vi "Delete Room.vi"(8 "error in (no error)":errorcluster, 10 "Room GUID":string, 11 "Room-API in":refnum<class "Room-API.lvclass">) -> (0 "error out":errorcluster, 2 "deleted?":bool, 3 "Room-API out":refnum<class "Room-API.lvclass">)   [LabVIEW 2020, in "Room-API.lvclass"]
uses:
  Room-API.lvclass
  Room-API.lvclass/Room-API.ctl
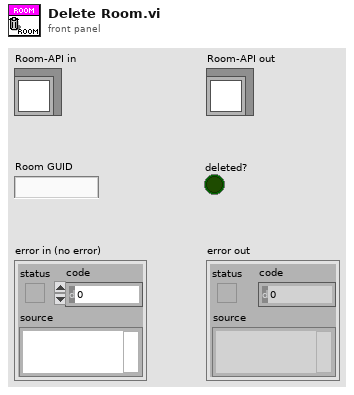
[diagram p1: front panel]
types:
  T1 = typedef "Room-API.lvclass/Single Room.ctl" = cluster{"name":string, "temperature_humidity":string[], "bond":string[], "hue":string[]}
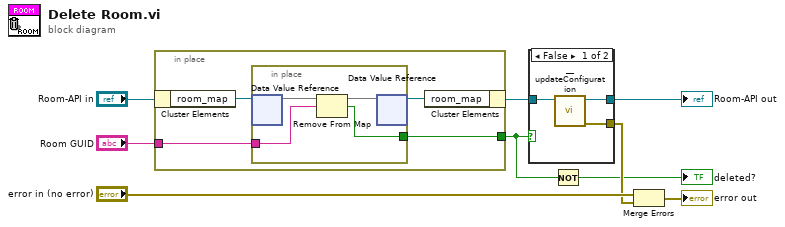
[diagram p0: block diagram]
diagram:
  n1 = in-place {
    in-place-border: "Room GUID" -> [w12]
    in-place-border: [w10] -> w2
    n2 = in-place-cluster #1("Room-API in") -> ("room_map"=w13:refnum<data-value>)
    n3 = in-place {
      in-place-border: w12 -> [w16]
      in-place-border: [w14] -> w10
      n4 = in-place-dvr #2(w13) -> (w17:map{string, T1})  [unwired: 1 out]
      n5 = Remove From Map(10:w16, 11:w17) -> (2:w14:bool, 3:w15:map{string, T1})  [unwired: 1 out]
      n6 = in-place-dvr #2(w15) -> (w11:refnum<data-value>)  [unwired: 1 out]
    }
    n7 = in-place-cluster #1("room_map"=w11) -> (w6:refnum<class "Room-API.lvclass">)
  }
  n8 = case shown="False" w2 {
    tunnel: w6 -> [w20 w21]
    tunnel: [w19 w21] -> w4
    tunnel: [w18 _] -> w5
    frame False {
      n9 = call "__updateConfiguration.vi"("Room-API in"=w20) -> ("error out"=w18:errorcluster, "Room-API out"=w19:refnum<class "Room-API.lvclass">)  [unwired: 9 in]
    }
    frame True {
    }
  }
  "Room-API out" <- w4
  n10 = Not(x=w2) -> (.not. x?=→"deleted?":bool)
  n11 = Merge Errors("error in (no error)", w5) -> (→"error out":errorcluster)
